vi "Log紀錄.vi"(5 "State":T1(ring)=enum."Standard", 7 "Activate?":bool, 9 "Application Directory":path, 10 "內容":string, 11 "Enum":enum16{"Create", "Write", "Close"}(ring)) -> ()   [LabVIEW 2016]
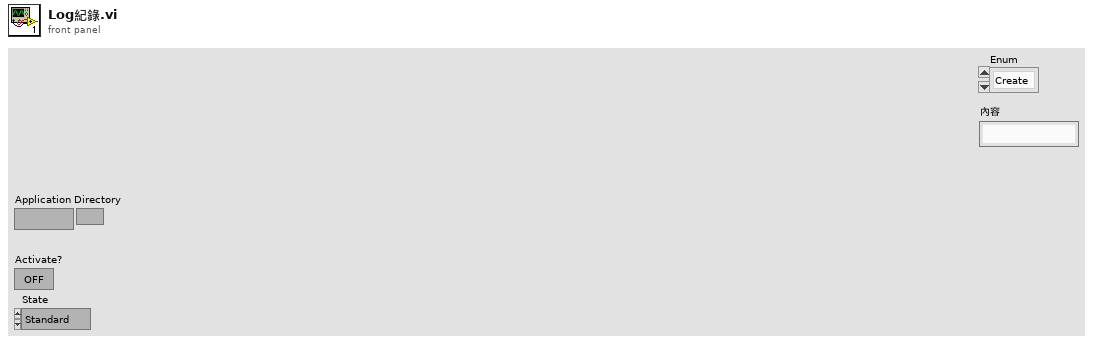
[diagram p1: front panel]
types:
  T1 = enum32{"Invalid", "Standard", "Closed", "Hidden", "Minimized", "Maximized"}
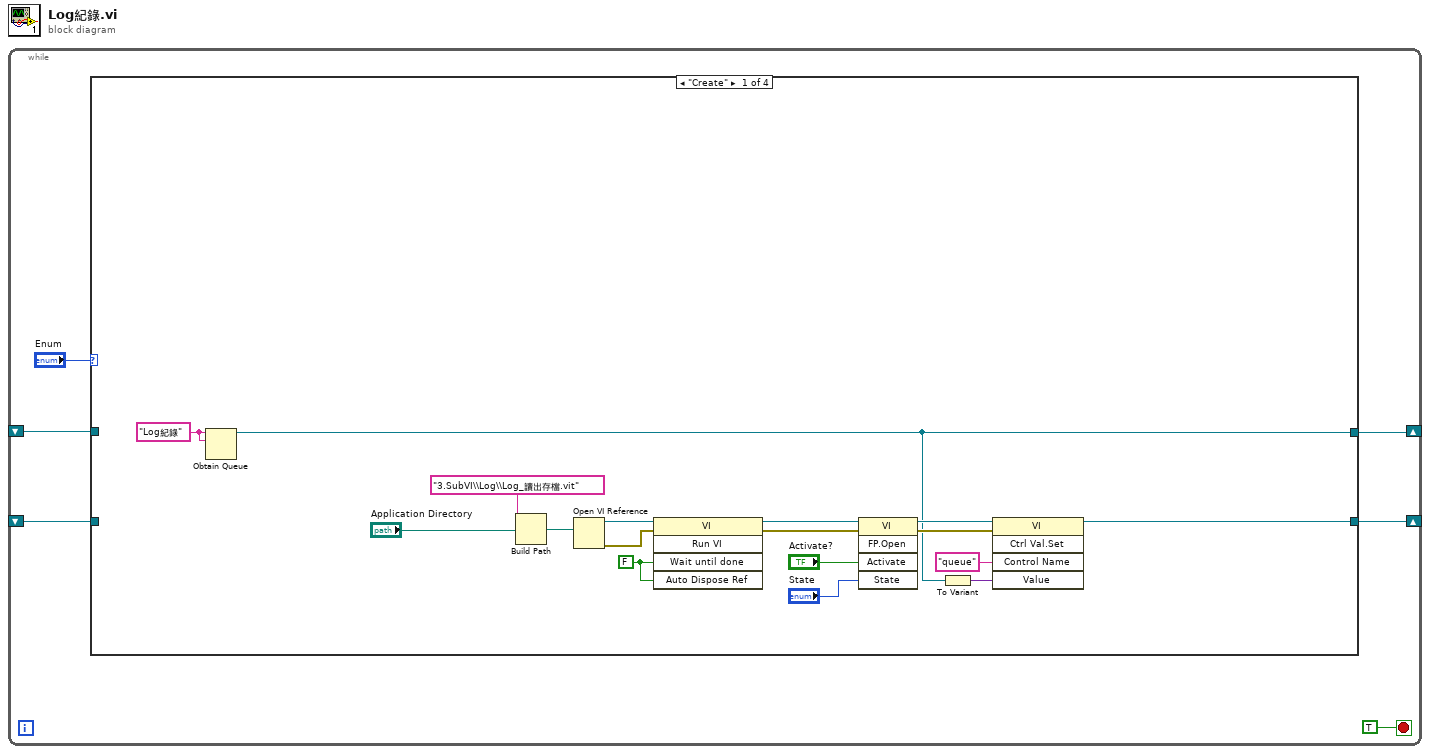
[diagram p0: block diagram]
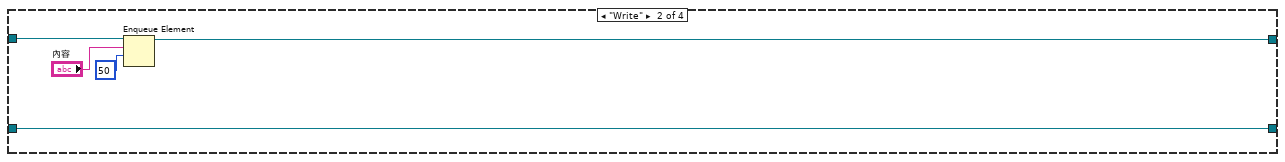
[diagram p2: hidden frame]
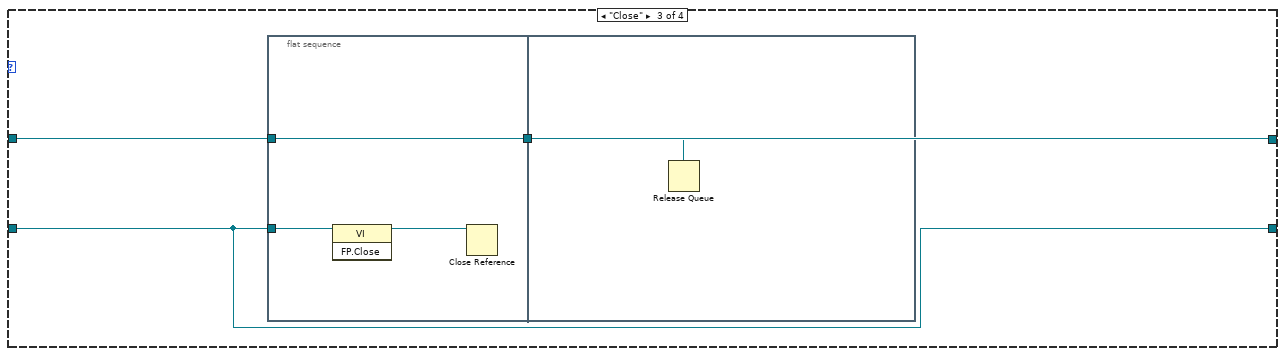
[diagram p3: hidden frame]
diagram:
  n1 = while {
    shift-right: [w4] -> _
    shift-left: _ -> [w3]
    shift-right: [w2] -> _
    shift-left: _ -> [w1]
    stop <- TRUE stop-if-true
    n2 = case shown="\"Create\"" "Enum" {
      tunnel: [w8 w25 w31 w37] -> w4
      tunnel: w3 -> [_ w28 w31 w37]
      tunnel: [w7 w24 w29 w36] -> w2
      tunnel: w1 -> [_ w24 w29 w36]
      frame "Create" {
        w20 = FALSE ("Wait until done")
        w23 = "Log紀錄" ("name (unnamed)")
        n3 = Obtain Queue(name (unnamed)=w23, element data type=w23) -> (queue out=w8:refnum<queue>)  [unwired: 3 in, 2 out]
        n4 = Build Path(base path="Application Directory", name or relative path="3.SubVI\\Log\\Log_讀出存檔.vit") -> (appended path=w14:path)
        n5 = Open VI Reference(vi path=w14) -> (vi reference=w10:refnum<vi>, error out=w21:errorcluster)  [unwired: 5 in]
        n6 = invoke class="VI" method="Run VI"(reference=w10, error in=w21, "Wait until done"=w20, "Auto Dispose Ref"=w20) -> (reference out=w18:refnum<vi>, error out=w19:errorcluster)  [unwired: 1 in, 3 out]
        n7 = invoke class="VI" method="FP.Open"(reference=w18, error in=w19, "Activate"="Activate?", "State"="State") -> (reference out=w22:refnum<vi>, error out=w12:errorcluster)  [unwired: 1 in, 3 out]
        n8 = To Variant(anything=w8) -> (Variant=w11:variant)
        n9 = invoke class="VI" method="Ctrl Val.Set"(reference=w22, error in=w12, "Control Name"="queue", "Value"=w11) -> (reference out=w7:refnum<vi>)  [unwired: 1 in, 4 out]
      }
      frame "Write" {
        n10 = Enqueue Element(queue=w28, element="內容", timeout in ms (-1)=50) -> (queue out=w25:refnum<queue>)  [unwired: 1 in, 2 out]
      }
      frame "Close" {
        n11 = flat-sequence {
          tunnel: w31 -> [w34]
          tunnel: [w34] -> w30
          tunnel: w29 -> [w33]
          tunnel: w30 -> [w35]
          frame #0 {
            n12 = invoke class="VI" method="FP.Close"(reference=w33) -> (reference out=w32:refnum<vi>)  [unwired: 2 in, 2 out]
            n13 = Close Reference(reference=w32) -> ()  [unwired: 1 in, 1 out]
          }
          frame #1 {
            n14 = Release Queue(queue=w35) -> ()  [unwired: 2 in, 3 out]
          }
        }
      }
      frame Default {
      }
    }
  }
